vi "DetectAndConnectCamera.vi"(8 "error in (no error)":errorcluster, 11 "Config In":T1 {"Hardware Configuration"."Lasers Configuration"."SettingValues"."785 Power" format="%.1f"; "Hardware Configuration"."Lasers Configuration"."SettingValues"."647 Power" format="%.1f"; "Hardware Configuration"."Lasers Configuration"."SettingValues"."561 Power" format="%.1f"; "Hardware Configuration"."Lasers Configuration"."SettingValues"."532 Power" format="%.1f"; "Hardware Configuration"."Lasers Configuration"."SettingValues"."488 Power" format="%.1f"; "Hardware Configuration"."Lasers Configuration"."SettingValues"."405 Power" format="%.1f"}) -> (0 "error out":errorcluster, 3 "Config Out":T1 {"Hardware Configuration"."Lasers Configuration"."SettingValues"."785 Power" format="%.1f"; "Hardware Configuration"."Lasers Configuration"."SettingValues"."647 Power" format="%.1f"; "Hardware Configuration"."Lasers Configuration"."SettingValues"."561 Power" format="%.1f"; "Hardware Configuration"."Lasers Configuration"."SettingValues"."532 Power" format="%.1f"; "Hardware Configuration"."Lasers Configuration"."SettingValues"."488 Power" format="%.1f"; "Hardware Configuration"."Lasers Configuration"."SettingValues"."405 Power" format="%.1f"})   [LabVIEW 2019]
uses:
  Settings/Settings.ctl
  Support/Hardware Configuration.ctl
  Support/Camera Configuration.ctl
  E:/DevHardSoftware/MMicroscopy/HardwareAdapter/Camera/Dependencies/PVCamNET.dll
  Dependencies/PVCamNET.dll
  <vilib>/userdefined/High Color/IMAQdx.ctl
  E:/DevHardSoftware/MMicroscopy/HardwareAdapter/Lasers/Dependencies/Oxxius_Boxx.dll
  Lasers/Dependencies/Oxxius_Boxx.dll
  Logging/Logging Configuration.ctl
  controls/UI Configuration.ctl
  Logging/Logging.lvlib
  Settings/Settings.lvlib
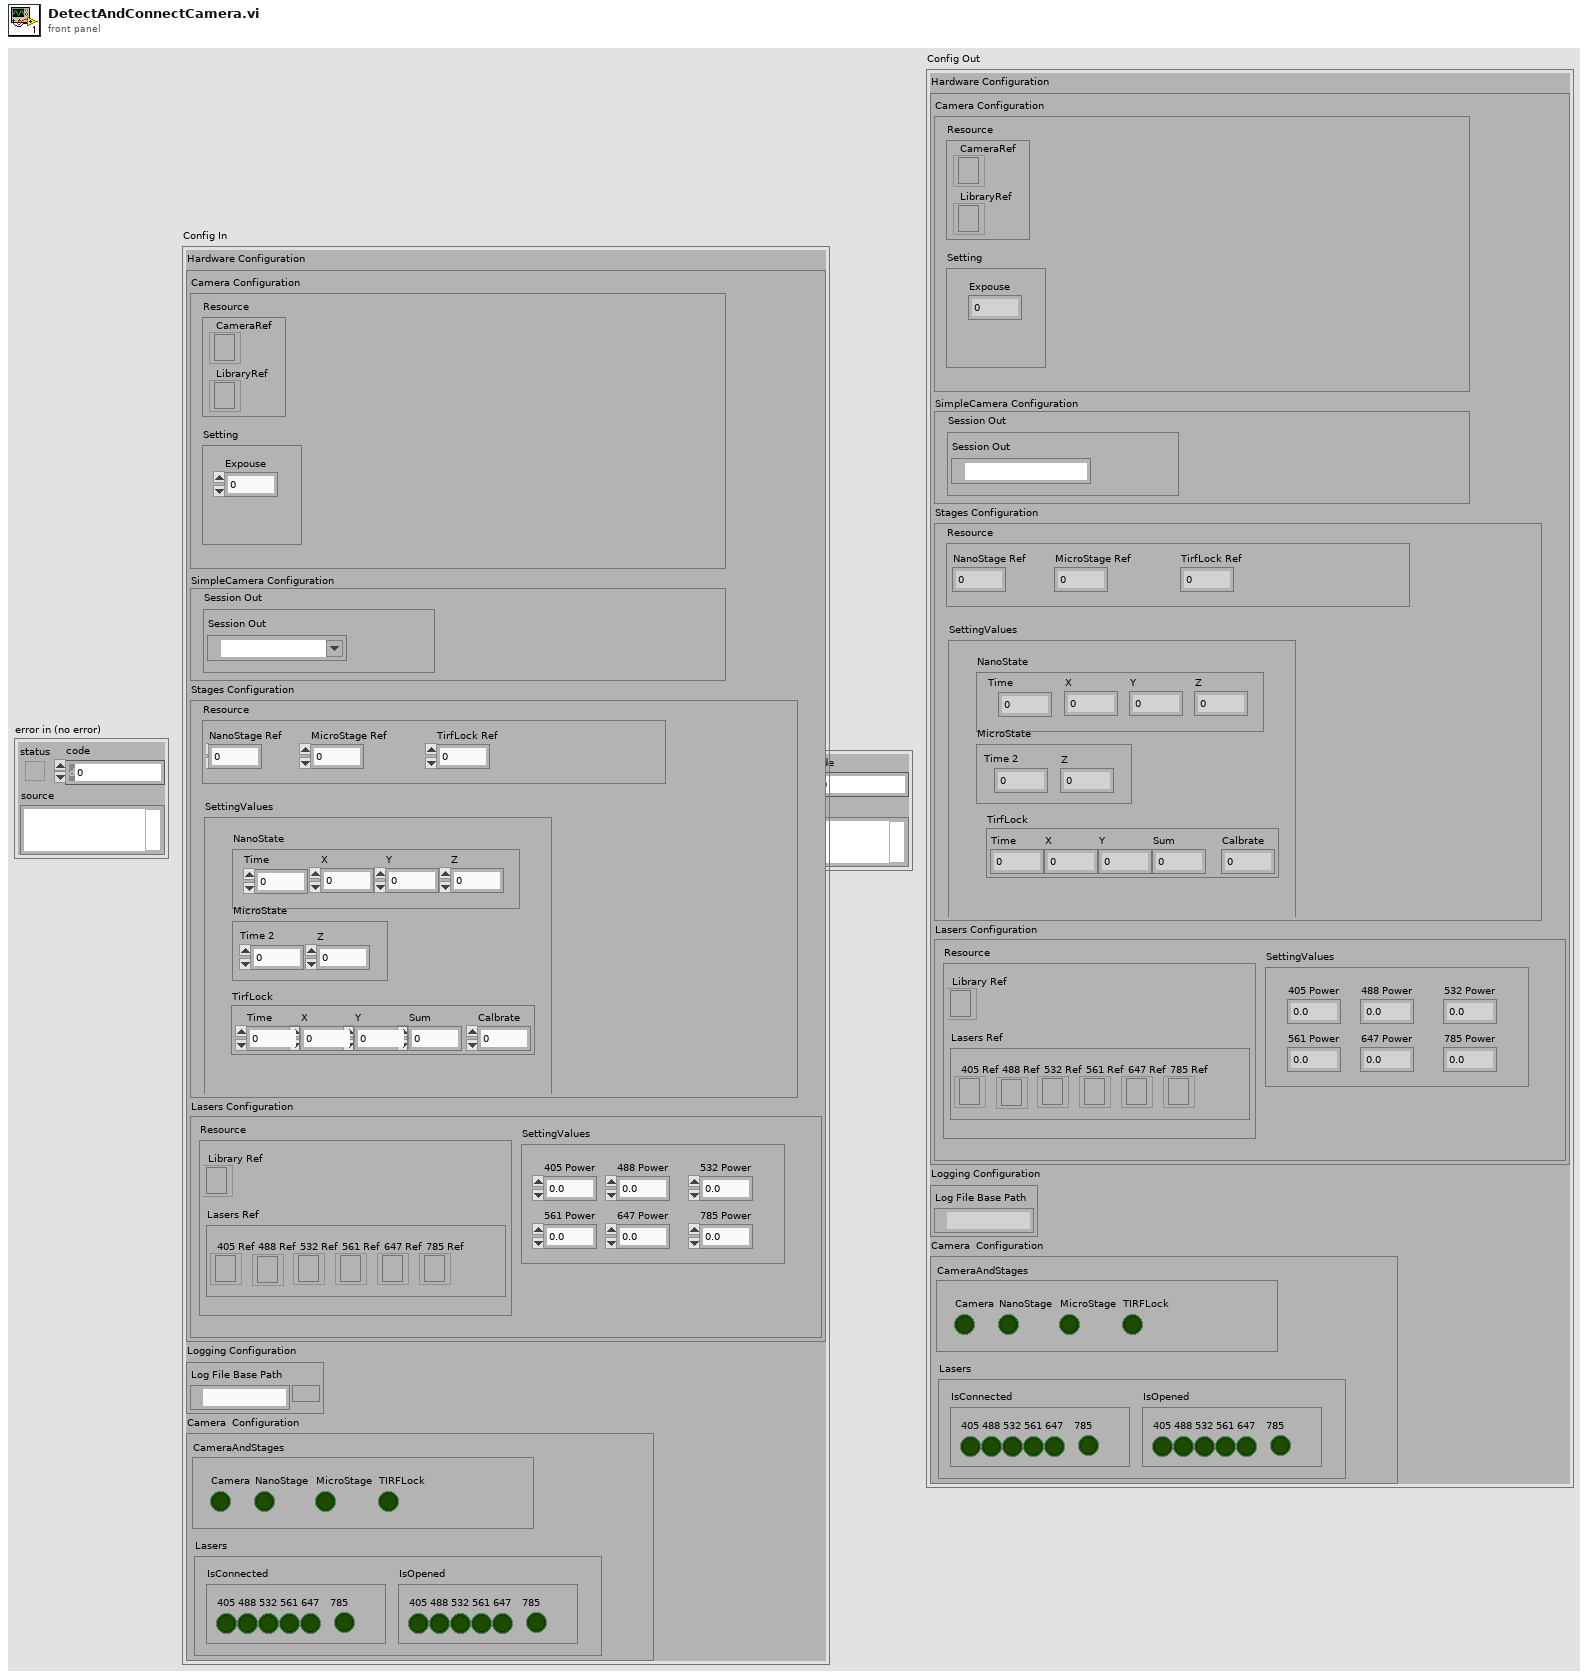
[diagram p1: front panel]
types:
  T1 = typedef "Settings.lvlib/Settings.ctl" = cluster{"Hardware Configuration":T2, "Logging Configuration":T5, "HardWare Status":cluster{"CameraAndStages":T6, "Lasers":cluster{"IsConnected":cluster{"405":bool, "488":bool, "532":bool, "561":bool, "647":bool, "785":bool}, "IsOpened":cluster{"405":bool, "488":bool, "532":bool, "561":bool, "647":bool, "785":bool}}}}
  T2 = typedef "Hardware Configuration.ctl" = cluster{"Camera Configuration":T3, "SimpleCamera Configuration":cluster{"Resource":cluster{"Session Out":T4}}, "Stages Configuration":cluster{"Resource":cluster{"NanoStage Ref":i32, "MicroStage Ref":i32, "TirfLock Ref":i32}, "SettingValues":cluster{"NanoState":cluster{"Time":dbl, "X":dbl, "Y":dbl, "Z":dbl}, "MicroState":cluster{"Time 2":dbl, "Z":dbl}, "TirfLock":cluster{"Time":dbl, "X":dbl, "Y":dbl, "Sum":dbl, "Calbrate":dbl}}}, "Lasers Configuration":cluster{"SettingValues":cluster{"405 Power":sgl, "488 Power":sgl, "532 Power":sgl, "561 Power":sgl, "647 Power":sgl, "785 Power":sgl}, "Resource":cluster{"Library Ref":refnum<k24>, "Lasers Ref":cluster{"405 Ref":refnum<k24>, "488 Ref":refnum<k24>, "532 Ref":refnum<k24>, "561 Ref":refnum<k24>, "647 Ref":refnum<k24>, "785 Ref":refnum<k24>}}}}
  T3 = typedef "Camera Configuration.ctl" = cluster{"Resource":cluster{"CameraRef":refnum<k24>, "LibraryRef":refnum<k24>}, "Setting":cluster{"Expouse":dbl}}
  T4 = typedef "IMAQdx.ctl" = refnum<k21>
  T5 = typedef "Logging.lvlib/Logging Configuration.ctl" = cluster{"Log File Base Path":path}
  T6 = typedef "UI Configuration.ctl" = cluster{"Camera":bool, "NanoStage":bool, "MicroStage":bool, "TIRFLock":bool}
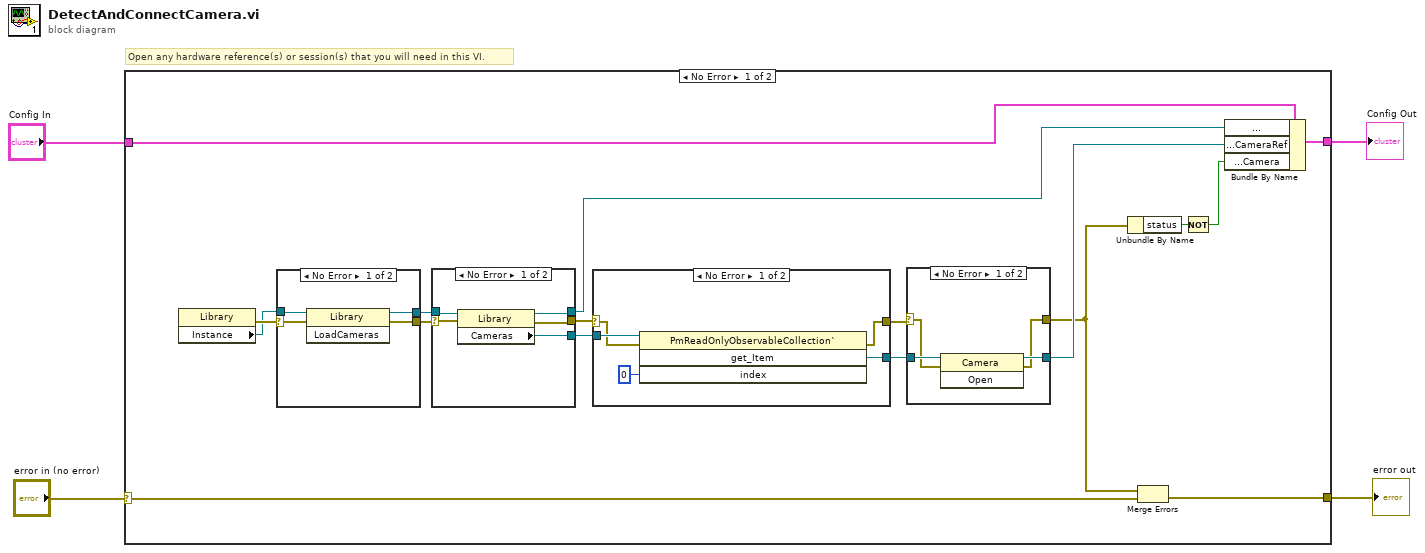
[diagram p0: block diagram]
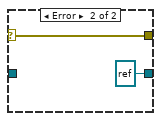
[diagram p2: hidden frame]
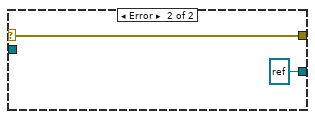
[diagram p3: hidden frame]
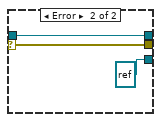
[diagram p4: hidden frame]
diagram:
  # "Open any hardware reference(s) or session(s) that you will need in this VI."
  n1 = case shown="No Error" "error in (no error)" {
    selector: "error in (no error)" -> [w21 w49]
    tunnel: [w20 w49] -> w3
    tunnel: "Config In" -> [w11 w50]
    tunnel: [w10 w50] -> w1
    frame No Error {
      n2 = property class="Library"() -> (error out=w19:errorcluster, "Instance"=w16:refnum<k24>)  [unwired: 2 in, 1 out]
      n3 = case shown="No Error" w19 {
        selector: w19 -> [w44 w48]
        tunnel: [w45 w48] -> w17
        tunnel: [w46 w47] -> w18
        tunnel: w16 -> [w43 w47]
        frame No Error {
          n4 = invoke class="Library" method="LoadCameras"(reference=w43, error in=w44) -> (reference out=w46:refnum<k24>, error out=w45:errorcluster)  [unwired: 1 in, 1 out]
        }
        frame Error {
        }
      }
      n5 = case shown="No Error" w17 {
        selector: w17 -> [w39 w42]
        tunnel: [w36 w42] -> w13
        tunnel: w18 -> [w38 w41]
        tunnel: [w37 w41] -> w9
        tunnel: [w35 refnum<k24> refnum ("Cameras")] -> w15
        frame No Error {
          n6 = property class="Library"(reference=w38, error in=w39) -> (reference out=w37:refnum<k24>, error out=w36:errorcluster, "Cameras"=w35:refnum<k24>)
        }
        frame Error {
        }
      }
      n7 = case shown="No Error" w13 {
        selector: w13 -> [w29 w34]
        tunnel: w15 -> [w32 _]
        tunnel: [w30 refnum<k24> refnum ("get_Item")] -> w14
        tunnel: [w28 w34] -> w12
        frame No Error {
          n8 = invoke class="PmReadOnlyObservableCollection`" method="get_Item"(reference=w32, error in=w29, "index"=0) -> (error out=w28:errorcluster, "get_Item"=w30:refnum<k24>)  [unwired: 1 in, 2 out]
        }
        frame Error {
        }
      }
      n9 = case shown="No Error" w12 {
        selector: w12 -> [w23 w27]
        tunnel: [w22 w27] -> w7
        tunnel: w14 -> [w25 _]
        tunnel: [w24 refnum<k24> refnum ("get_Item")] -> w8
        frame No Error {
          n10 = invoke class="Camera" method="Open"(reference=w25, error in=w23) -> (reference out=w24:refnum<k24>, error out=w22:errorcluster)  [unwired: 1 in, 1 out]
        }
        frame Error {
        }
      }
      n11 = Unbundle By Name(w7) -> ("status"=w6:bool)
      n12 = Merge Errors(w7, w21) -> (w20:errorcluster)
      n13 = Not(x=w6) -> (.not. x?=w5:bool)
      n14 = Bundle By Name(cluster=w11, "Hardware Configuration.Camera Configuration.Resource.LibraryRef"=w9, "Hardware Configuration.Camera Configuration.Resource.CameraRef"=w8, "HardWare Status.CameraAndStages.Camera"=w5) -> (w10:T1)
    }
    frame Error {
    }
  }
  "error out" <- w3
  "Config Out" <- w1
